vi "Send Message (Batch).vi"(8 "error in (no error)":errorcluster, 9 "Delay Seconds":i32[](array[numeric]), 10 "Message Bodies":string[](array[string]), 11 "SQS in":refnum<class "NI_AWS_SQS.lvclass">) -> (0 "error out":errorcluster, 1 "Message Body MD5s":string[](array[string]), 2 "Message IDs":string[](array[string]), 3 "SQS out":refnum<class "NI_AWS_SQS.lvclass">)   [LabVIEW 2015, in "NI_AWS_SQS.lvclass"]
uses:
  NI_AWS_SQS.lvclass
  Core/Name Value Pair.ctl
  Core/Request Options.ctl
  NI_AWS_SQS.lvclass/NI_AWS_SQS.ctl
  Read Account Number.vi
  Read Name.vi
  <vilib>/Utility/error.llb/Error Cluster From Error Code.vi
  <vilib>/ErrorRing/Error Ring.xnode
  Core/NI_AWS_Core.lvclass
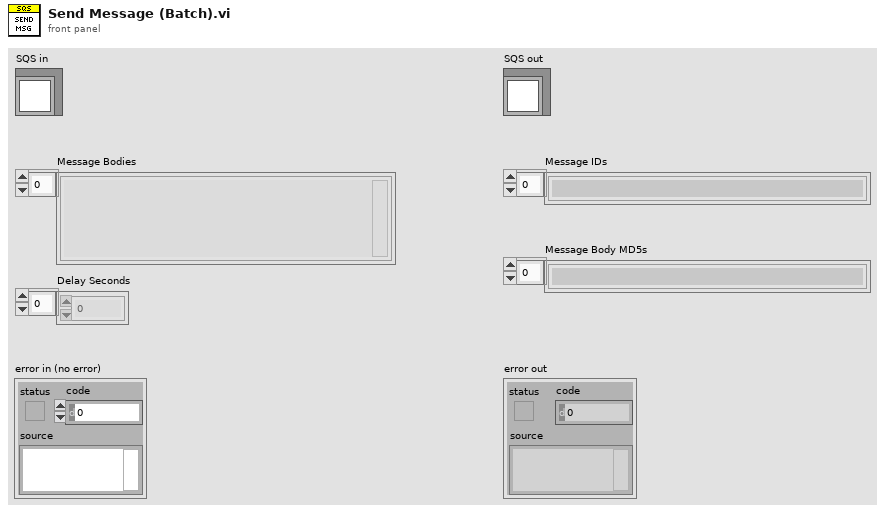
[diagram p1: front panel]
types:
  T1 = typedef "NI_AWS_Core.lvclass/Request Options.ctl" = cluster{"request headers":T2[], "request parameters":T2[], "request body":string}
  T2 = typedef "NI_AWS_Core.lvclass/Name Value Pair.ctl" = cluster{"name":string, "value":string}
  T3 = typedef "NI_AWS_Core.lvclass/Response.ctl" = cluster{"Headers":string, "Body":string}
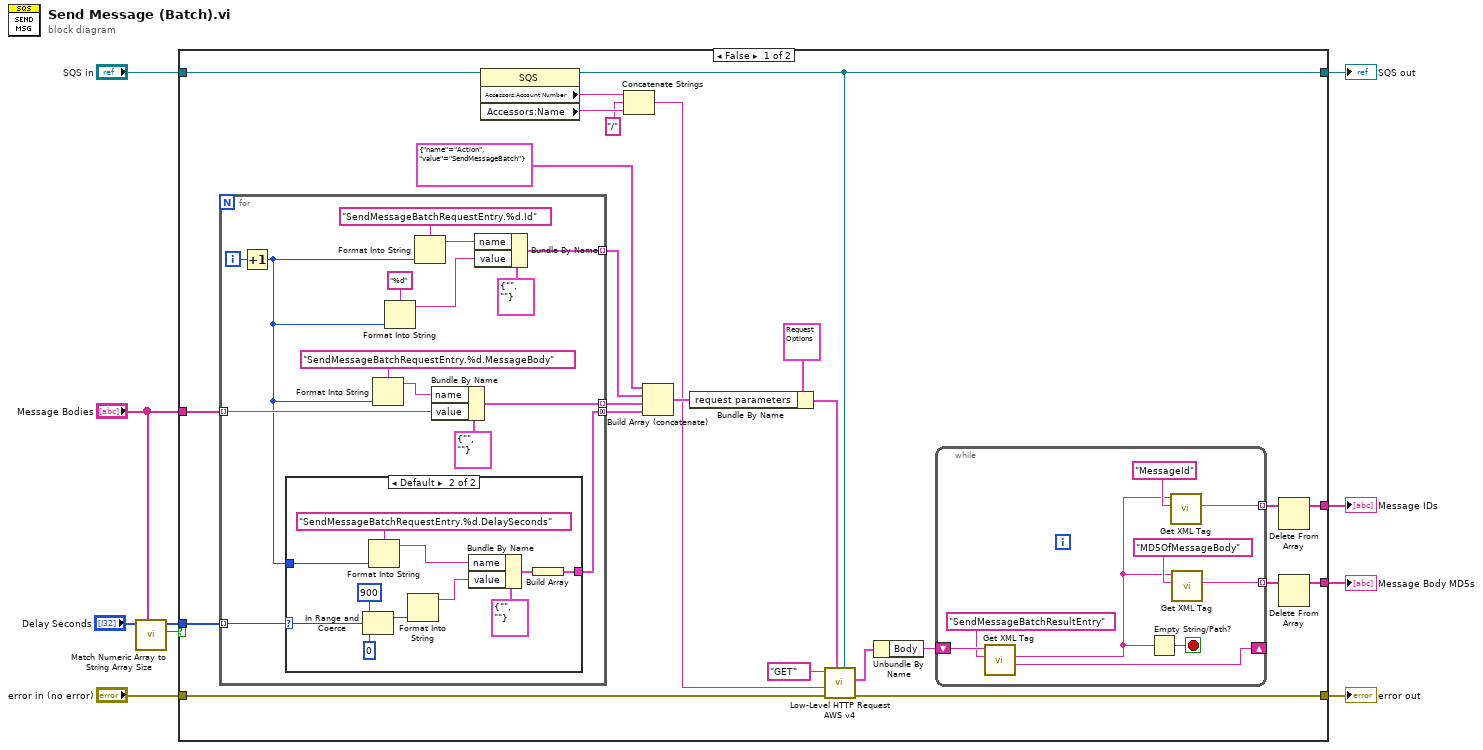
[diagram p0: block diagram]
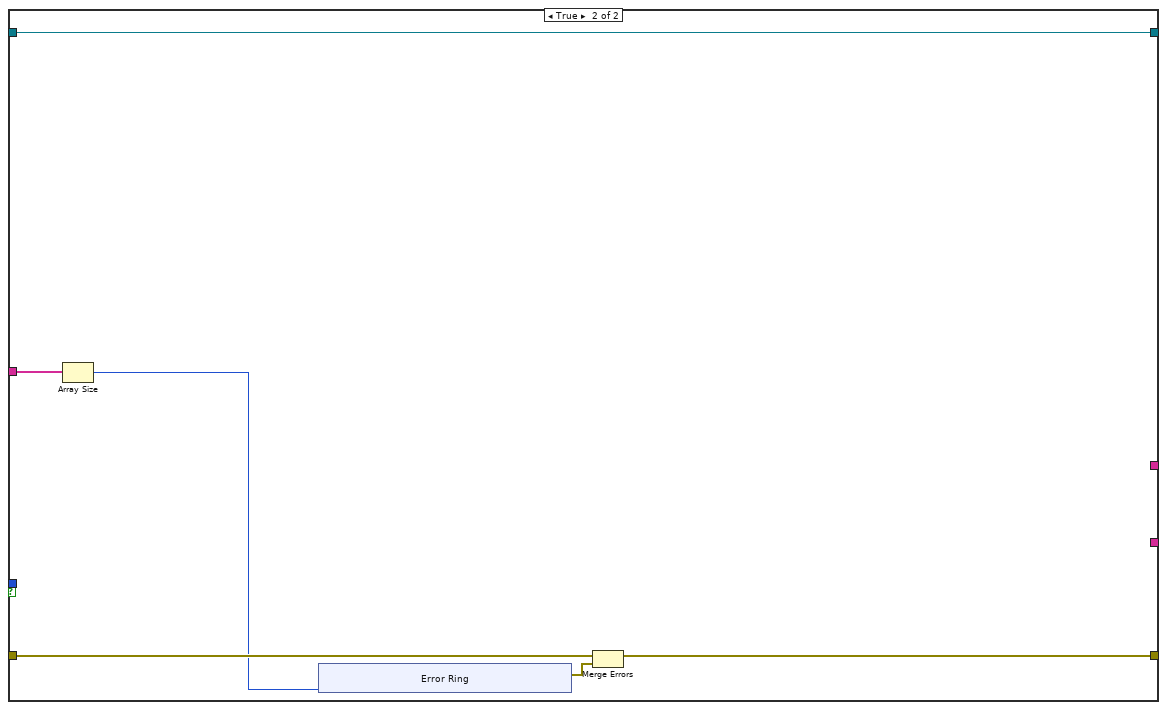
[diagram p3: hidden frame]
diagram:
  n1 = call "Match Numeric Array to String Array Size.vi"("String Array"="Message Bodies", "Numeric Array in"="Delay Seconds") -> ("Exceeded Max Size"=w1:bool, "Numeric Array out"=w5:i32[])  [unwired: 8 in]
  n2 = case shown="False" w1 {
    tunnel: "error in (no error)" -> [w34 w75]
    tunnel: [w33 w74] -> w9
    tunnel: "SQS in" -> [w32 w73]
    tunnel: [w27 w73] -> w7
    tunnel: w5 -> [w18 _]
    tunnel: "Message Bodies" -> [w17 w71]
    tunnel: [w12 _] -> w3
    tunnel: [w11 _] -> w2
    frame False {
      n3 = for {
        tunnel: [w48] -> w22 mode=indexing
        tunnel: [w35] -> w21 mode=concatenating
        tunnel: w17 -> [w37] mode=indexing
        tunnel: w18 -> [w47] mode=indexing
        tunnel: [w44] -> w19 mode=indexing
        i -> [w45]
        n4 = Increment(x=w45) -> (x+1=w36:i32)
        n5 = case shown="Default" w47 {
          selector: w47 -> [_ w54]
          tunnel: w36 -> [_ w51]
          tunnel: [_ w50] -> w35
          frame 0 {
          }
          frame Default {
            n6 = In Range and Coerce(upper limit=900, x=w54, lower limit=0) -> (coerced(x)=w56:i32)  [unwired: 1 out]
            n7 = Format Into String(format string="SendMessageBatchRequestEntry.%d.DelaySeconds" ("name"), w51) -> (resulting string=w52:string)  [unwired: 2 in, 1 out]
            n8 = Format Into String(w56) -> (resulting string=w55:string)  [unwired: 3 in, 1 out]
            n9 = Bundle By Name(cluster=T2 {"name"="", "value"=""} ("element"), "name"=w52, "value"=w55) -> (w59:T2)
            n10 = Build Array(w59) -> (w50:T2[])
          }
        }
        n11 = Format Into String(format string="SendMessageBatchRequestEntry.%d.MessageBody" ("name"), w36) -> (resulting string=w38:string)  [unwired: 2 in, 1 out]
        n12 = Format Into String(format string="%d", w36) -> (resulting string=w40:string)  [unwired: 2 in, 1 out]
        n13 = Format Into String(format string="SendMessageBatchRequestEntry.%d.Id" ("name"), w36) -> (resulting string=w43:string)  [unwired: 2 in, 1 out]
        n14 = Bundle By Name(cluster=T2 {"name"="", "value"=""} ("element"), "name"=w38, "value"=w37) -> (w48:T2)
        n15 = Bundle By Name(cluster=T2 {"name"="", "value"=""} ("element"), "name"=w43, "value"=w40) -> (w44:T2)
      }
      n16 = property class="SQS"(reference=w32) -> (reference out=w27:refnum<class "NI_AWS_SQS.lvclass">, "Accessors:Account Number"=w26:string, "Accessors:Name"=w25:string)  [unwired: 1 in, 1 out]
      n17 = Concatenate Strings(w26, "/", w25) -> (w23:string)
      n18 = Build Array (concatenate)(T2 {"name"="Action", "value"="SendMessageBatch"} ("Cluster"), w19, w22, w21) -> (w28:T2[])
      n19 = Bundle By Name(cluster=T1 {"request headers"=[], "request parameters"=[{"name"="Action", "value"="ListQueues"}], "request body"=""} ("Request Options"), "request parameters"=w28) -> (w29:T1)
      n20 = call "Low-Level HTTP Request AWS v4.vi"("AWS Core"=w27, "Request Options"=w29, "error in (no error)"=w34, "URL Suffix"=w23, "HTTP-Verb"="GET") -> ("error out"=w33:errorcluster, "Response"=w16:T3)  [unwired: 4 in, 1 out]
      n21 = Unbundle By Name(w16) -> ("Body"=w15:string)
      n22 = while {
        shift-right: [w68] -> _
        shift-left: w15 -> [w69]
        tunnel: [w62] -> w14 mode=indexing
        tunnel: [w61] -> w13 mode=indexing
        stop <- w67 stop-if-true
        n23 = call "Get XML Tag.vi"("Tag name"="SendMessageBatchResultEntry", "XML String in"=w69) -> ("Remaining string"=w68:string, "Tag value"=w63:string)  [unwired: 5 in, 3 out]
        n24 = Empty String/Path?(string/path=w63) -> (empty?=w67:bool)
        n25 = call "Get XML Tag.vi"("Tag name"="MessageId", "XML String in"=w63) -> ("Tag value"=w62:string)  [unwired: 5 in, 4 out]
        n26 = call "Get XML Tag.vi"("Tag name"="MD5OfMessageBody", "XML String in"=w63) -> ("Tag value"=w61:string)  [unwired: 5 in, 4 out]
      }
      n27 = Delete From Array(array=w14) -> (array with subset deleted=w12:string[])  [unwired: 2 in, 1 out]
      n28 = Delete From Array(array=w13) -> (array with subset deleted=w11:string[])  [unwired: 2 in, 1 out]
    }
    frame True {
      n29 = Array Size(array=w71) -> (size(s)=w70:i32)
      n30 = xnode "Error Ring"("parameter 0"=w70) -> ("error out"=w72:errorcluster)
      n31 = Merge Errors(w75, w72) -> (w74:errorcluster)
    }
  }
  "error out" <- w9
  "SQS out" <- w7
  "Message IDs" <- w3
  "Message Body MD5s" <- w2
